vi "Get Gyro.vi"() -> (2 "Angle":dbl)   [LabVIEW 2014]
uses:
  Robot Global Data.vi
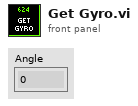
[diagram p1: front panel]
types:
  T1 = typedef "WPI_GyroDevRef.ctl" = cluster{"DevStatus":errorcluster, "Analog Module":T2, "Analog Channel":T3, "Offset":dbl, "Gain (VoltsPerDegree/Second)":dbl}
  T2 = typedef "FPGA_TypedefAnalogModule.ctl" = enum16{"Controller 1"}
  T3 = typedef "FPGA_AIChannel.ctl" = enum8{"AI 0", "AI 1", "AI 2", "AI 3", "AI MXP 0", "AI MXP 1", "AI MXP 2", "AI MXP 3", "Invalid"}
  T4 = typedef "IMU Data.ctl" = cluster{"Pitch":sgl, "Roll":sgl, "Yaw":sgl}
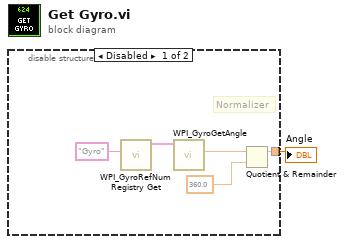
[diagram p0: block diagram]
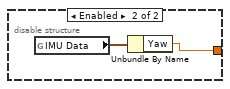
[diagram p2: hidden frame]
diagram:
  n1 = disable-structure shown="Disabled" {
    disable-tunnel: [w2 w7] -> w1
    frame Disabled {
      # "Normalizer"
      n2 = call <vilib>:"WPI_GyroRefNum Registry Get.vi"("refnum name"="Gyro") -> ("GyroDevRef"=w5:T1)  [unwired: 9 in, 1 out]
      n3 = call <vilib>:"WPI_GyroGetAngle.vi"("GyroDevRef"=w5) -> ("Angle"=w4:dbl)  [unwired: 7 in, 3 out]
      n4 = Quotient & Remainder(x=w4, y=360.0) -> (x-y*floor(x/y)=w2:dbl)  [unwired: 1 out]
    }
    frame Enabled {
      n5 = global read "Robot Global Data.vi" "IMU Data"() -> (w8:T4)
      n6 = Unbundle By Name(w8) -> ("Yaw"=w7:sgl)
    }
  }
  "Angle" <- w1
